vi "KepcoDCPwr Reset.vi"(0 "VISA Session":refnum<visa-resource-name>, 5 "Model In":string, 7 "channel name (\"\")":string="\"\"", 11 "error in (no error)":errorcluster {"code" format="%.0x"}) -> (4 "VISA Session Out":refnum<visa-resource-name>, 6 "Model Out":string, 8 "channel name out (\"\")":string="\"\"" caption="channel name Out (\"\")", 15 "error out":errorcluster {"code" format="%.0x"})   [LabVIEW 2020]
doc: "This VI resets the instrument to a known state and sends initialization commands to the instrument. The initialization commands set instrument settings such as Headers Off, Short Command form, and Data Transfer Binary to the state necessary for the operation of the instrument driver."
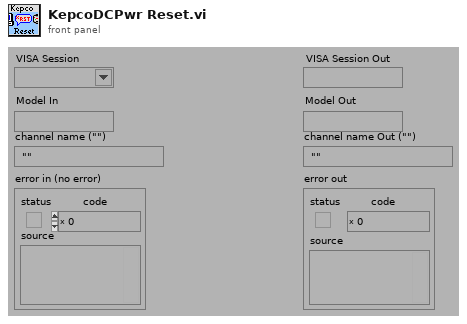
[diagram p1: front panel]
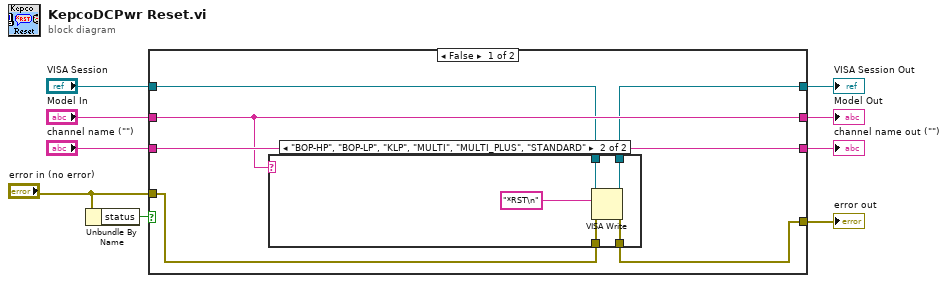
[diagram p0: block diagram]
diagram:
  n1 = Unbundle By Name("error in (no error)") -> ("status"=w8:bool)
  n2 = case shown="False" w8 {
    tunnel: [w11 w26] -> w9
    tunnel: "error in (no error)" -> [w10 w26]
    tunnel: [w12 w25] -> w1
    tunnel: "VISA Session" -> [w13 w25]
    tunnel: [w14 w24] -> w2
    tunnel: "Model In" -> [w14 w24]
    tunnel: [w15 w23] -> w3
    tunnel: "channel name (\"\")" -> [w15 w23]
    frame False {
      n3 = case shown="\"BOP-HP\", \"BOP-LP\", \"KLP\", \"MULTI\", \"MULTI_PLUS\", \"STANDARD\"" w14 {
        tunnel: w10 -> [w17 w22]
        tunnel: [w17 w21] -> w11
        tunnel: w13 -> [w16 w20]
        tunnel: [w16 w19] -> w12
        frame "", Default {
        }
        frame "BOP-HP", "BOP-LP", "KLP", "MULTI", "MULTI_PLUS", "STANDARD" {
          n4 = VISA Write(VISA resource name=w20, write buffer="*RST\n", error in (no error)=w22) -> (VISA resource name out=w19:refnum<visa-resource-name>, error out=w21:errorcluster)  [unwired: 1 out]
        }
      }
    }
    frame True {
    }
  }
  "error out" <- w9
  "channel name out (\"\")" <- w3
  "Model Out" <- w2
  "VISA Session Out" <- w1
